vi "Main Initialize.vi"(8 "Parameters in":T2={"J1939 XNET Settings"={"XNET Database"="", "XNET Cluster"="", "CAN Port"="", "Baud rate [Bd]"=0, "J1939 Network Address"=0, "Name"=0, "Termination"=1, "Incoming Rate"=100, "Outcoming Rate"=100}, "Incoming Single Point Configuraiton"={"Incoming Single Point Frame"={"ID"=[], "Conversion"=[], "Channel Array Positions"=[], "Frame Length"=[]}, "Channel Pairs"={"Chan Refs"=[], "Previous Chan Values"=[]}, "Read FIFO"=refnum}, "Outgoing Cyclic Configuraiton"={"Outgoing Cyclic Frame"={"ID"=[], "Conversion"=[], "Channel Array Positions"=[], "Frame Length"=[], "Transmit Propreties"=[]}, "Channel Pairs"={"Block Data Refs"=[], "Previous Chan Values"=[]}, "Write FIFO"=refnum, "Write Decimation"=1}} {"Outgoing Cyclic Configuraiton"."Channel Pairs"."Block Data Refs"."Data Reference" format="%.0x"; "Outgoing Cyclic Configuraiton"."Outgoing Cyclic Frame"."Transmit Propreties"."Transmit Time" format="%#_p"; "J1939 XNET Settings"."Termination" items=["Off", "On"]; "Incoming Single Point Configuraiton"."Channel Pairs"."Chan Refs" format="%.0x"}, 9 "Name in":string, 10 "Parent VI Ref":refnum<vi>, 11 "Parent":string) -> (0 "error out":errorcluster, 2 "Notification":bool, 3 "J1939 Main Configuration":T1={"Parameters"={"J1939 XNET Settings"={"XNET Database"="", "XNET Cluster"="", "CAN Port"="", "Baud rate [Bd]"=0, "J1939 Network Address"=0, "Name"=0, "Termination"=1, "Incoming Rate"=100, "Outcoming Rate"=100}, "Incoming Single Point Configuraiton"={"Incoming Single Point Frame"={"ID"=[], "Conversion"=[], "Channel Array Positions"=[], "Frame Length"=[]}, "Channel Pairs"={"Chan Refs"=[], "Previous Chan Values"=[]}, "Read FIFO"=refnum}, "Outgoing Cyclic Configuraiton"={"Outgoing Cyclic Frame"={"ID"=[], "Conversion"=[], "Channel Array Positions"=[], "Frame Length"=[], "Transmit Propreties"=[]}, "Channel Pairs"={"Block Data Refs"=[], "Previous Chan Values"=[]}, "Write FIFO"=refnum, "Write Decimation"=1}}, "Name"="", "J1939 Cluster"={"Processed Incoming"=refnum, "Current Device Address"=0, "Processed Outgoing"=refnum, "Process Outgoing"=refnum, "Name"=0}, "References"={"BAM Buffer"=refnum, "CM Buffer"=refnum, "CM Gen"=refnum, "BAM Gen"=refnum, "Address Claims"=refnum, "RQST"=refnum}, "StopRef"=refnum, "Frame In"="", "Frame Out"="", "Incoming Timeout"=0, "Outgoing Timeout"=0, "Listener ID"=refnum, "Parent VI Ref"=refnum, "Data Ref"=refnum, "Scale Ref"=refnum, "Incoming Direct Access"={"Offset"=0, "Length"=0}, "Outgoing Direct Access"={"Offset"=0, "Length"=0}, "vi reference"=refnum, "Name and Address"=""} {"Parameters"."Outgoing Cyclic Configuraiton"."Channel Pairs"."Block Data Refs"."Data Reference" format="%.0x"; "Parameters"."Outgoing Cyclic Configuraiton"."Outgoing Cyclic Frame"."Transmit Propreties"."Transmit Time" format="%#_p"; "Parameters"."J1939 XNET Settings"."Termination" items=["Off", "On"]; "Parameters"."Incoming Single Point Configuraiton"."Channel Pairs"."Chan Refs" format="%.0x"})   [LabVIEW 2013, in "J1939 Addon Engine.lvlib"]
uses:
  J1939 Addon Engine.lvlib
  Types/Process Parameters.ctl
  Shared/Types/XNET Settings.ctl
  Types/Incoming Single Point Configuration.ctl
  Types/Incoming Single Point Frame Pairs.ctl
  Types/Incoming Single Point Channel Pairs.ctl
  <vilib>/NI Veristand/Custom Device API/Data Reference.ctl
  Types/Outgoing Cyclic Configuration.ctl
  Types/Outgoing Cyclic Frame Pairs.ctl
  Shared/Types/XNET Frame Event Properties.ctl
  Types/Outgoing Cyclic Channel Pairs.ctl
  <vilib>/NI Veristand/Custom Device API/Block Data Reference.ctl
  Types/Configuration Cluster.ctl
  Shared/J1939 Multi Packet Frame/Types/Setup Information Cluster.ctl
  <vilib>/xnet/xnet.llb/XNET Frame CAN.ctl
  <vilib>/xnet/xnet.llb/XNET Frame Type CAN.ctl
  Shared/J1939 Utilities/Types/CAN Outgoing Message Cluster.ctl
  Shared/J1939 Multi Packet Frame/Types/TP List References.ctl
  Shared/J1939 Multi Packet Frame/Types/BAM Buffer Connections List_Ref.ctl
  Shared/J1939 Multi Packet Frame/Types/Connection Mode Generation Connection Ref.ctl
  Shared/J1939 Multi Packet Frame/Types/BAM Generation Connections List_Ref.ctl
  Shared/J1939 Multi Packet Frame/Types/Address Table Reference.ctl
  Shared/J1939 Multi Packet Frame/Types/RQST Lookup Table Reference.ctl
  Stop FG/Stop Global Ref.ctl
  Types/Data Lookup Table Reference.ctl
  Types/Conversion Lookup Table Reference.ctl
  Shared/J1939 Multi Packet Frame/Types/RQST Comm Lookup Table_Ref.ctl
  <vilib>/xnet/xnet.llb/XNET Create Session (Frame Output Stream).vi
  <vilib>/xnet/xnet.llb/XNET Create Session (Frame Input Stream).vi
  Inline Async API/Inline Async API.lvlib
  Error Handling API/Error Handling API.lvlib
  Stop FG/Stop FG.lvlib
  <resource>/objmgr/xnet.rc
  Shared/J1939 Addon Shared.lvlib
  <vilib>/NI Veristand/Custom Device API/Custom Device API.lvlib
  Shared/J1939 Utilities/J1939 Utilities.lvlib
  <vilib>/NI Veristand/Custom Device Tools/Custom Device Utility Library/Custom Device Utility Library.lvlib
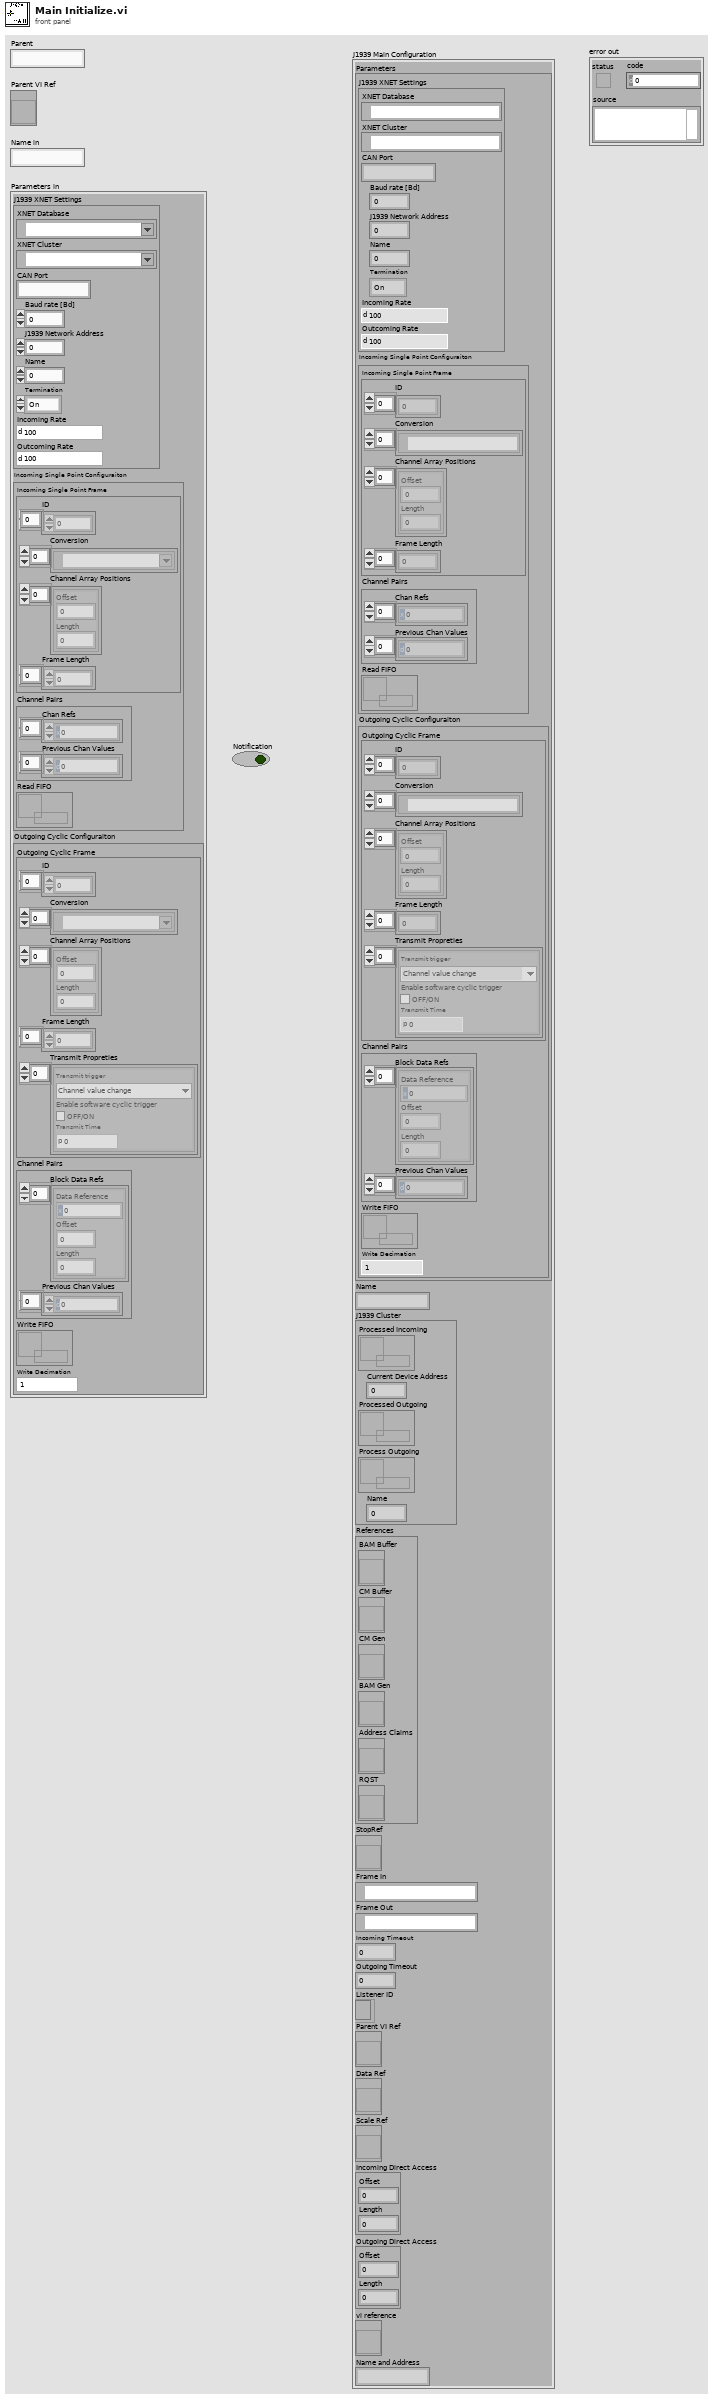
[diagram p1: front panel]
types:
  T1 = typedef "J1939 Addon Engine.lvlib/Configuration Cluster.ctl" = cluster{"Parameters":T2, "Name":string, "J1939 Cluster":T13, "References":T14, "StopRef":T20, "Frame In":refnum<k21>, "Frame Out":refnum<k21>, "Incoming Timeout":u32, "Outgoing Timeout":u32, "Listener ID":refnum<k5>, "Parent VI Ref":refnum<vi>, "Data Ref":T21, "Scale Ref":T22, "Incoming Direct Access":cluster{"Offset":u32, "Length":u32}, "Outgoing Direct Access":cluster{"Offset":u32, "Length":u32}, "vi reference":T23, "Name and Address":string}
  T2 = typedef "J1939 Addon Engine.lvlib/Process Parameters.ctl" = cluster{"J1939 XNET Settings":T3, "Incoming Single Point Configuraiton":T4, "Outgoing Cyclic Configuraiton":T8}
  T3 = typedef "J1939 Addon Shared.lvlib/XNET Settings.ctl" = cluster{"XNET Database":refnum<k21>, "XNET Cluster":refnum<k21>, "CAN Port":string, "Baud rate [Bd]":u32, "J1939 Network Address":u8, "Name":u64, "Termination":u32, "Incoming Rate":u32, "Outcoming Rate":u32}
  T4 = typedef "J1939 Addon Engine.lvlib/Incoming Single Point Configuration.ctl" = cluster{"Incoming Single Point Frame":T5, "Channel Pairs":T6, "Read FIFO":refnum<k33>}
  T5 = typedef "J1939 Addon Engine.lvlib/Incoming Single Point Frame Pairs.ctl" = cluster{"ID":u32[], "Conversion":refnum<k21>[], "Channel Array Positions":cluster{"Offset":u32, "Length":u32}[], "Frame Length":u32[]}
  T6 = typedef "J1939 Addon Engine.lvlib/Incoming Single Point Channel Pairs.ctl" = cluster{"Chan Refs":T7[], "Previous Chan Values":dbl[]}
  T7 = typedef "Custom Device API.lvlib/Data Reference.ctl" = i32
  T8 = typedef "J1939 Addon Engine.lvlib/Outgoing Cyclic Configuration.ctl" = cluster{"Outgoing Cyclic Frame":T9, "Channel Pairs":T11, "Write FIFO":refnum<k33>, "Write Decimation":u32}
  T9 = typedef "J1939 Addon Engine.lvlib/Outgoing Cyclic Frame Pairs.ctl" = cluster{"ID":u32[], "Conversion":refnum<k21>[], "Channel Array Positions":cluster{"Offset":u32, "Length":u32}[], "Frame Length":u32[], "Transmit Propreties":T10[]}
  T10 = typedef "J1939 Addon Shared.lvlib/XNET Frame Event Properties.ctl" = cluster{"Transmit trigger":enum16{"Channel value change"}, "Enable software cyclic trigger":bool, "Transmit Time":dbl}
  T11 = typedef "J1939 Addon Engine.lvlib/Outgoing Cyclic Channel Pairs.ctl" = cluster{"Block Data Refs":T12[], "Previous Chan Values":dbl[]}
  T12 = typedef "Custom Device API.lvlib/Block Data Reference.ctl" = cluster{"Data Reference":T7, "Offset":i32, "Length":i32}
  T13 = typedef "J1939 Addon Engine.lvlib/Setup Information Cluster.ctl" = cluster{"Processed Incoming":refnum<queue>, "Current Device Address":u8, "Processed Outgoing":refnum<queue>, "Process Outgoing":refnum<queue>, "Name":u64}
  T14 = typedef "J1939 Addon Engine.lvlib/TP List References.ctl" = cluster{"BAM Buffer":T15, "CM Buffer":T15, "CM Gen":T16, "BAM Gen":T17, "Address Claims":T18, "RQST":T19}
  T15 = typedef "J1939 Addon Engine.lvlib/BAM Buffer Connections List_Ref.ctl" = refnum<vi>
  T16 = typedef "J1939 Addon Engine.lvlib/Connection Mode Generation Connection Ref.ctl" = refnum<vi>
  T17 = typedef "J1939 Addon Engine.lvlib/BAM Generation Connections List_Ref.ctl" = refnum<vi>
  T18 = typedef "J1939 Addon Engine.lvlib/Address Table Reference.ctl" = refnum<vi>
  T19 = typedef "J1939 Addon Engine.lvlib/RQST Lookup Table Reference.ctl" = refnum<vi>
  T20 = typedef "J1939 Addon Engine.lvlib/Stop FG.lvlib/Stop Global Ref.ctl" = refnum<vi>
  T21 = typedef "J1939 Addon Engine.lvlib/Data Lookup Table Reference.ctl" = refnum<vi>
  T22 = typedef "J1939 Addon Engine.lvlib/Conversion Lookup Table Reference.ctl" = refnum<vi>
  T23 = typedef "J1939 Addon Engine.lvlib/RQST Comm Lookup Table_Ref.ctl" = refnum<vi>
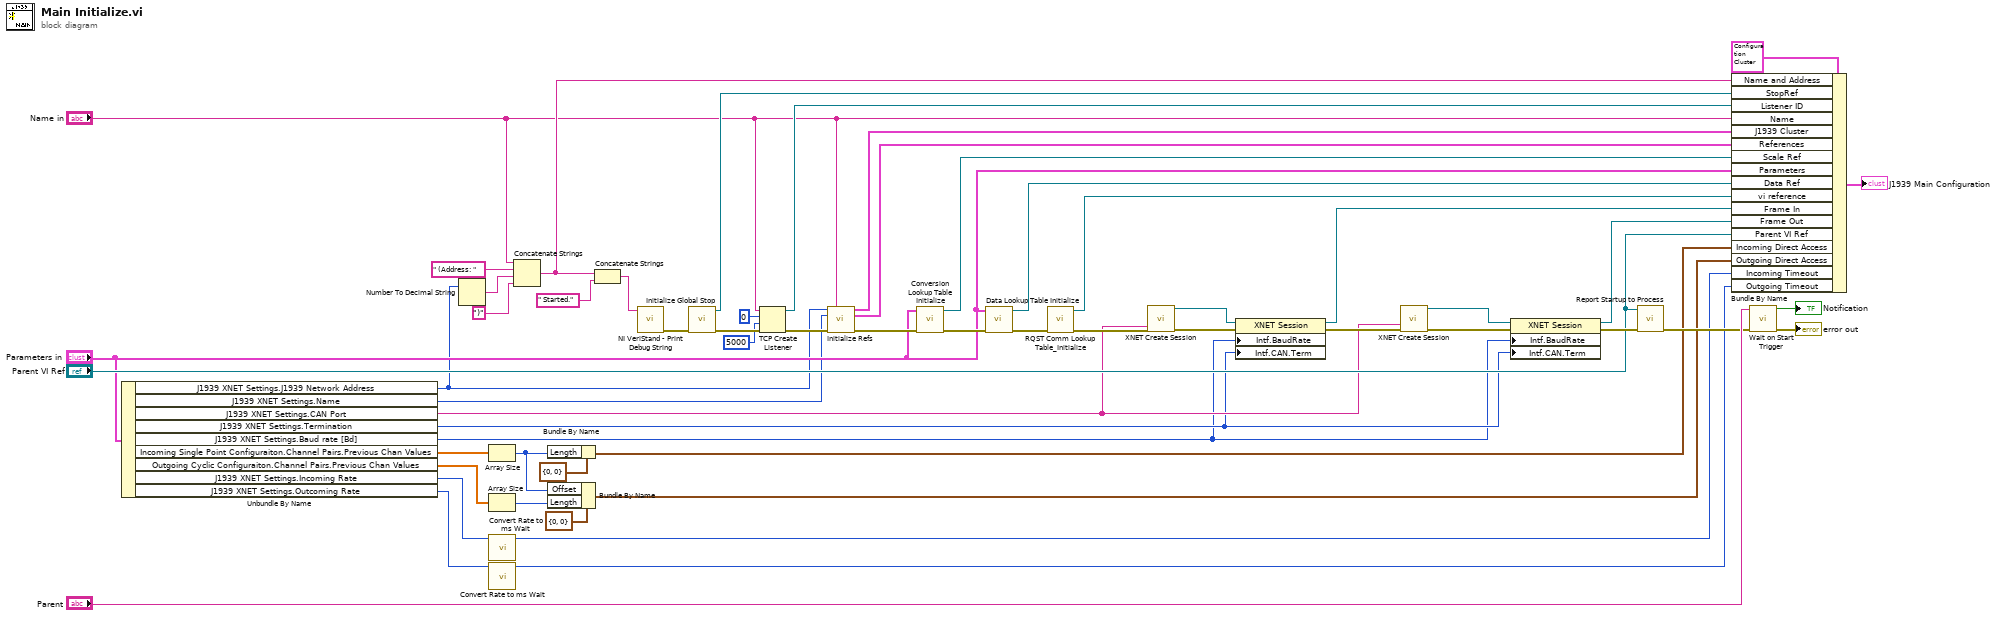
[diagram p0: block diagram]
diagram:
  n1 = Unbundle By Name("Parameters in") -> ("J1939 XNET Settings.J1939 Network Address"=w3:u8, "J1939 XNET Settings.Name"=w2:u64, "J1939 XNET Settings.CAN Port"=w15:string, "J1939 XNET Settings.Termination"=w14:u32, "J1939 XNET Settings.Baud rate [Bd]"=w13:u32, "Incoming Single Point Configuraiton.Channel Pairs.Previous Chan Values"=w43:dbl[], "Outgoing Cyclic Configuraiton.Channel Pairs.Previous Chan Values"=w18:dbl[], "J1939 XNET Settings.Incoming Rate"=w16:u32, "J1939 XNET Settings.Outcoming Rate"=w17:u32)
  n2 = Number To Decimal String(number=w3) -> (decimal integer string=w1:string)  [unwired: 1 in]
  n3 = Array Size(array=w43) -> (size(s)=w41:i32)
  n4 = Array Size(array=w18) -> (size(s)=w42:i32)
  n5 = call "Convert Rate to ms Wait.vi"("x"=w16) -> ("x*y"=w11:u32)  [unwired: 10 in]
  n6 = call "Convert Rate to ms Wait.vi"("x"=w17) -> ("x*y"=w12:u32)  [unwired: 10 in]
  n7 = Concatenate Strings("Name in", " (Address: " ("string"), w1, ")" ("string")) -> (w30:string)
  n8 = Bundle By Name(cluster=cluster{"Offset":u32, "Length":u32} {"Offset"=0, "Length"=0} ("Direct Access"), "Length"=w41) -> (w9:cluster{"Offset":u32, "Length":u32})
  n9 = Bundle By Name(cluster=cluster{"Offset":u32, "Length":u32} {"Offset"=0, "Length"=0} ("Direct Access"), "Offset"=w41, "Length"=w42) -> (w10:cluster{"Offset":u32, "Length":u32})
  n10 = Concatenate Strings(w30, " Started." ("string")) -> (w5:string)
  n11 = call <vilib>:"NI VeriStand - Print Debug String.vi"("Message"=w5) -> ("error out"=w33:errorcluster)  [unwired: 10 in]
  n12 = call "Initialize Global Stop.vi"("error in (no error)"=w33) -> ("error out"=w51:errorcluster, "vi reference"=w26:T20)  [unwired: 9 in]
  n13 = TCP Create Listener(8:w51, 9:5000 ("timeout ms (25000)"), 10:u16 0 ("port"), 11:"Name in") -> (0:w50:errorcluster, 3:w29:refnum<k5>)  [unwired: 1 in, 1 out]
  n14 = call "Initialize Refs.vi"("Current Device Address"=w3, "Name"="Name in", "Device Name"=w2, "error in (no error)"=w50) -> ("J1939 Cluster"=w28:T13, "References"=w27:T14, "error out"=w35:errorcluster)  [unwired: 9 out]
  n15 = call "Conversion Lookup Table Initialize.vi"("error in (no error)"=w35, "J1939 Process Parameters"="Parameters in") -> ("error out"=w36:errorcluster, "vi reference"=w22:T22)  [unwired: 8 in]
  n16 = call "Data Lookup Table Initialize.vi"("error in (no error)"=w36, "J1939 Process Parameters"="Parameters in") -> ("error out"=w52:errorcluster, "vi reference"=w21:T21)  [unwired: 8 in]
  n17 = call "RQST Comm Lookup Table_Initialize.vi"("error in (no error)"=w52) -> ("error out"=w53:errorcluster, "vi reference"=w25:T23)  [unwired: 9 in]
  n18 = call-poly <vilib>:"XNET Create Session.vi"("interface"=w15, "error in (no error)"=w53) -> ("session out"=w55:refnum<k21>, "error out"=w54:errorcluster)  [unwired: 12 out]
  n19 = property class="XNET Session"(reference=w55, error in=w54, "Intf.BaudRate"=w13, "Intf.CAN.Term"=w14) -> (reference out=w24:refnum<k21>, error out=w38:errorcluster)
  n20 = call-poly <vilib>:"XNET Create Session.vi"("interface"=w15, "error in (no error)"=w38) -> ("session out"=w45:refnum<k21>, "error out"=w44:errorcluster)  [unwired: 12 out]
  n21 = property class="XNET Session"(reference=w45, error in=w44, "Intf.BaudRate"=w13, "Intf.CAN.Term"=w14) -> (reference out=w23:refnum<k21>, error out=w56:errorcluster)
  n22 = call "Report Startup to Process.vi"("Error"=w56, "This VI"="Parent VI Ref") -> ("error out"=w34:errorcluster)  [unwired: 9 in]
  n23 = Bundle By Name(cluster=T1 {"Parameters"={"J1939 XNET Settings"={"XNET Database"="", "XNET Cluster"="", "CAN Port"="", "Baud rate [Bd]"=0, "J1939 Network Address"=0, "Name"=0, "Termination"=1, "Incoming Rate"=100, "Outcoming Rate"=100}, "Incoming Single Point Configuraiton"={"Incoming Single Point Frame"={"ID"=[], "Conversion"=[], "Channel Array Positions"=[], "Frame Length"=[]}, "Channel Pairs"={"Chan Refs"=[], "Previous Chan Values"=[]}, "Read FIFO"=refnum}, "Outgoing Cyclic Configuraiton"={"Outgoing Cyclic Frame"={"ID"=[], "Conversion"=[], "Channel Array Positions"=[], "Frame Length"=[], "Transmit Propreties"=[]}, "Channel Pairs"={"Block Data Refs"=[], "Previous Chan Values"=[]}, "Write FIFO"=refnum, "Write Decimation"=1}}, "Name"="", "J1939 Cluster"={"Processed Incoming"=refnum, "Current Device Address"=0, "Processed Outgoing"=refnum, "Process Outgoing"=refnum, "Name"=0}, "References"={"BAM Buffer"=refnum, "CM Buffer"=refnum, "CM Gen"=refnum, "BAM Gen"=refnum, "Address Claims"=refnum, "RQST"=refnum}, "StopRef"=refnum, "Frame In"="", "Frame Out"="", "Incoming Timeout"=0, "Outgoing Timeout"=0, "Listener ID"=refnum, "Parent VI Ref"=refnum, "Data Ref"=refnum, "Scale Ref"=refnum, "Incoming Direct Access"={"Offset"=0, "Length"=0}, "Outgoing Direct Access"={"Offset"=0, "Length"=0}, "vi reference"=refnum, "Name and Address"=""} ("output cluster"), "Name and Address"=w30, "StopRef"=w26, "Listener ID"=w29, "Name"="Name in", "J1939 Cluster"=w28, "References"=w27, "Scale Ref"=w22, "Parameters"="Parameters in", "Data Ref"=w21, "vi reference"=w25, "Frame In"=w24, "Frame Out"=w23, "Parent VI Ref"="Parent VI Ref", "Incoming Direct Access"=w9, "Outgoing Direct Access"=w10, "Incoming Timeout"=w11, "Outgoing Timeout"=w12) -> (→"J1939 Main Configuration":T1)
  n24 = call "Wait on Start Trigger.vi"("error in (no error)"=w34, "Name"="Parent") -> ("error out"=→"error out":errorcluster, "notification"=→"Notification":bool)  [unwired: 8 in]
